vi "handle_websocket_connection.vi"(3 "log queue":refnum<queue>, 4 "remote port":u16, 5 "# conn.":refnum<data-value>, 6 "remote address":string, 7 "quit?":refnum<notifier>, 8 "error in (no error)":errorcluster, 9 "max payload bytes (5012)":i32=5012, 10 "WebSocket Connection Handler":refnum<class "WebSocket Connection Handler.lvclass">, 11 "TCP Network Connection in":refnum<k5>) -> (0 "error out":errorcluster)   [LabVIEW 2019, in "WebSocket Server Toolkit.lvlib"]
uses:
  WebSocket Server Toolkit.lvlib
  types/opcode.ctl
  types/status_code.ctl
  types/frame_data.ctl
  classes/WebSocket Connection Handler/WebSocket Connection Handler.lvclass
  classes/WebSocket Connection/WebSocket Connection.lvclass
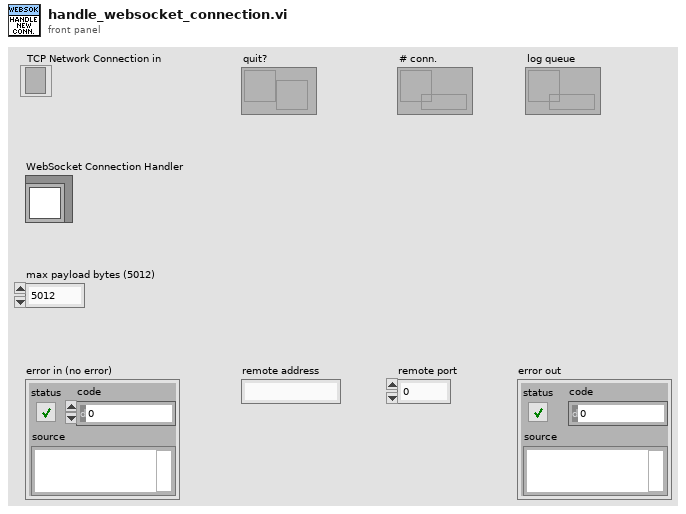
[diagram p1: front panel]
types:
  T1 = typedef "WebSocket Server Toolkit.lvlib/HTTP Request Method.ctl" = enum16{"GET", "HEAD", "POST", "PUT", "DELETE", "CONNECT", "OPTIONS", "TRACE", "PATCH"}
  T2 = typedef "WebSocket Server Toolkit.lvlib/HTTP Protocol Version.ctl" = enum16{"HTTP/0.9", "HTTP/1.0", "HTTP/1.1", "HTTP/2.0", "HTTP/3.0"}
  T3 = typedef "WebSocket Server Toolkit.lvlib/frame_data.ctl" = cluster{"binary?":bool, "frames":string[]}
  T4 = typedef "WebSocket Server Toolkit.lvlib/status_code.ctl" = u16
  T5 = typedef "WebSocket Server Toolkit.lvlib/opcode.ctl" = u8
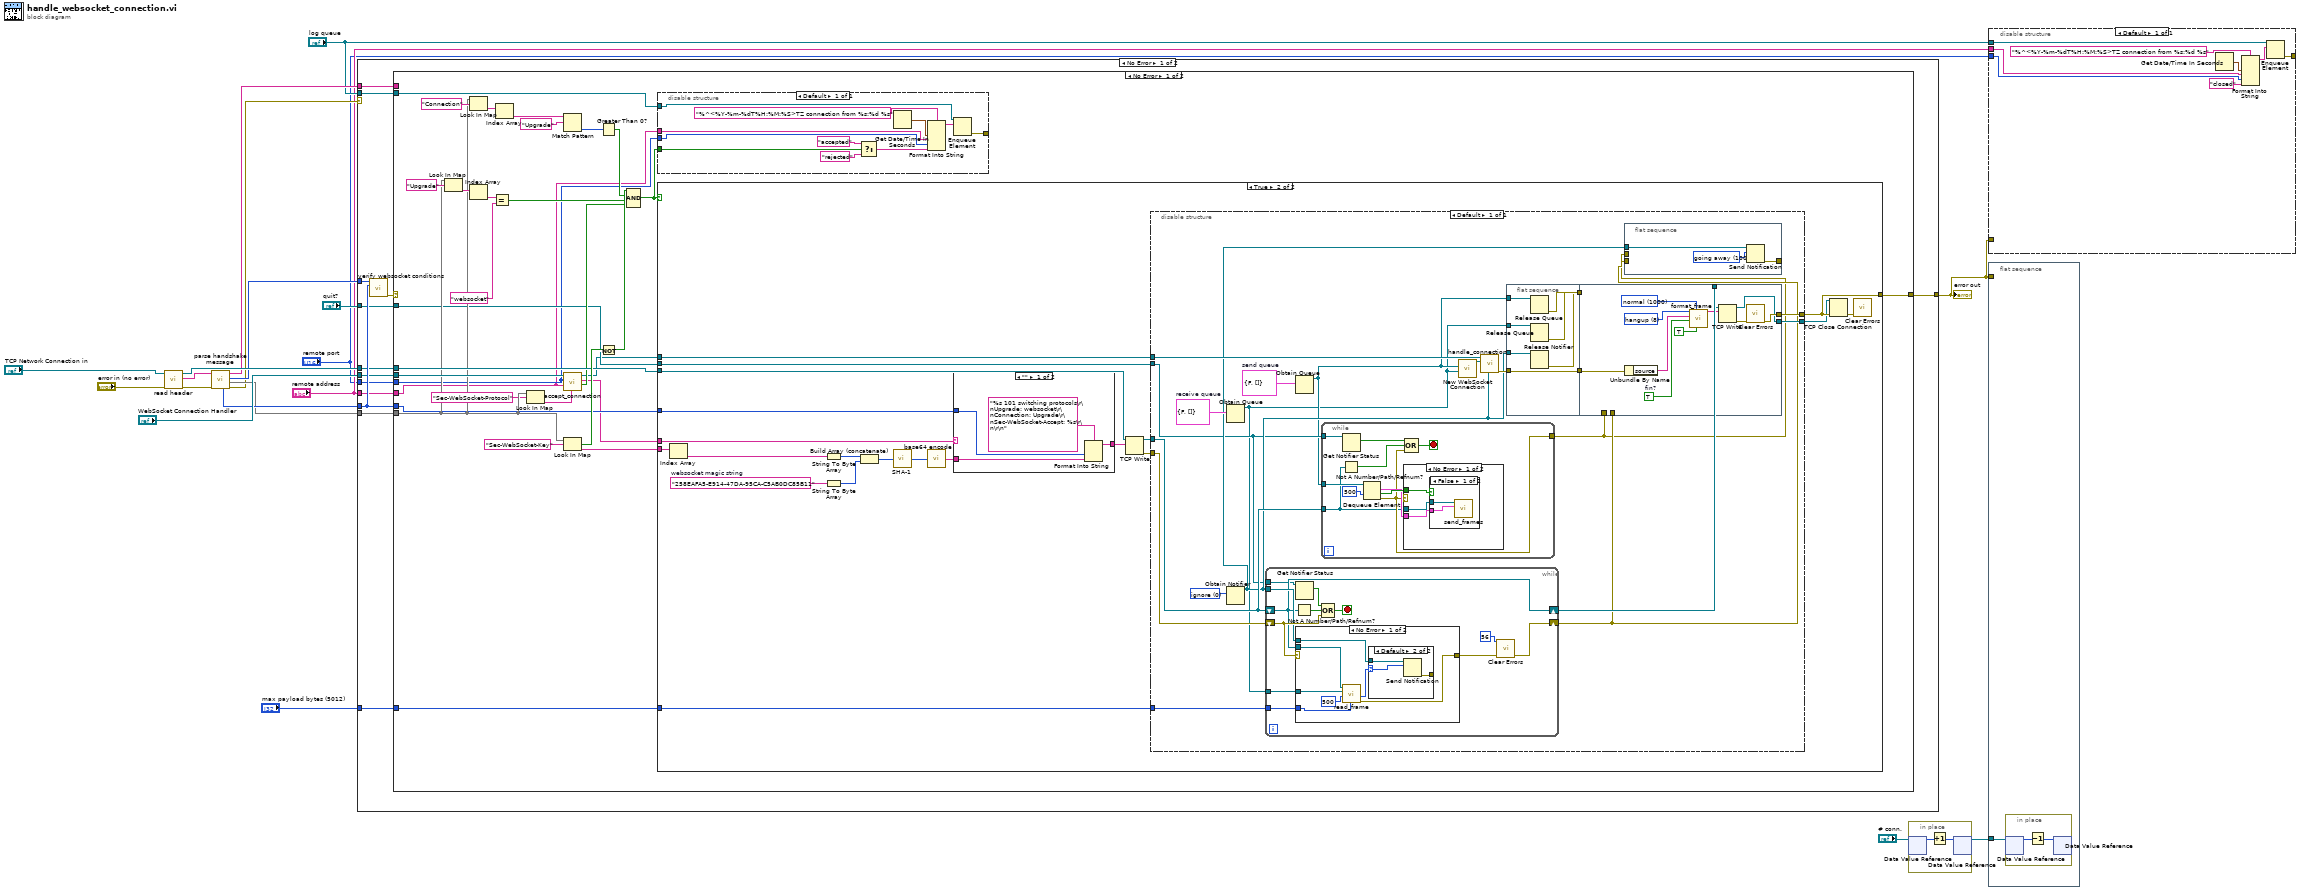
[diagram p0: block diagram]
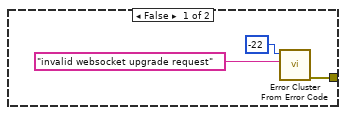
[diagram p2: hidden frame]
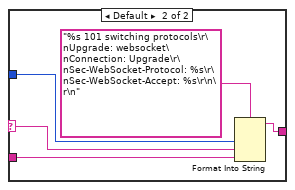
[diagram p7: hidden frame]
diagram:
  n1 = call "read header.vi"("error in (no error)"="error in (no error)", "TCP Network Connection in"="TCP Network Connection in") -> ("error out"=w11:errorcluster, "header content"=w12:string, "TCP Network Connection out"=w18:refnum<k5>)  [unwired: 7 in]
  n2 = call "parse handshake message.vi"("error in"=w11, "String"=w12) -> ("error out"=w13:errorcluster, "headers"=w16:map{string, string[]}, "HTTP method"=w15:T1, "URL"=w14:string, "HTTP protocol version"=w17:T2)  [unwired: 5 in]
  n3 = case shown="No Error" w13 {
    selector: w13 -> [_ w189]
    tunnel: w14 -> [w30 _]
    tunnel: w15 -> [w32 _]
    tunnel: w16 -> [w29 _]
    tunnel: w17 -> [w27 _]
    tunnel: [w28 w189] -> w1
    tunnel: w18 -> [w26 _]
    tunnel: "WebSocket Connection Handler" -> [w25 _]
    tunnel: "remote port" -> [w24 _]
    tunnel: "remote address" -> [w23 _]
    tunnel: "quit?" -> [w22 _]
    tunnel: "max payload bytes (5012)" -> [w21 _]
    tunnel: "log queue" -> [w20 _]
    frame No Error {
      n4 = call "verify websocket conditions.vi"("HTTP protocol version"=w27, "HTTP method"=w32) -> ("error out"=w31:errorcluster)  [unwired: 9 in]
      n5 = case shown="No Error" w31 {
        selector: w31 -> [_ w188]
        tunnel: w30 -> [_ _]
        tunnel: w29 -> [w48 _]
        tunnel: [w53 w188] -> w28
        tunnel: w27 -> [w52 _]
        tunnel: w26 -> [w51 _]
        tunnel: w25 -> [w50 _]
        tunnel: w24 -> [w36 _]
        tunnel: w23 -> [w35 _]
        tunnel: w22 -> [w43 _]
        tunnel: w21 -> [w41 _]
        tunnel: w20 -> [w34 _]
        frame No Error {
          n6 = Look In Map(map=w48, key="Upgrade") -> (value=w59:string[])  [unwired: 1 in, 1 out]
          n7 = Look In Map(map=w48, key="Connection") -> (value=w60:string[])  [unwired: 1 in, 1 out]
          n8 = Index Array(array=w59) -> (element=w49:string)  [unwired: 1 in]
          n9 = Equal?(x=w49, y="websocket") -> (x = y?=w55:bool)
          n10 = Index Array(array=w60) -> (element=w39:string)  [unwired: 1 in]
          n11 = Look In Map(map=w48, key="Sec-WebSocket-Protocol") -> (value=w46:string[])  [unwired: 1 in, 1 out]
          n12 = Match Pattern(string=w39, regular expression="Upgrade" ("y")) -> (offset past match=w38:i32)  [unwired: 1 in, 3 out]
          n13 = call-dynamic "accept_connection.vi"("Sec-WebSocket-Protocol"=w46, "remote address"=w35, "remote port"=w36, "WebSocket Connection Handler in"=w50) -> ("accept connection?"=w45:bool, "Sec-WebSocket-Protocol accepted"=w44:string, "WebSocket Connection Handler out"=w42:refnum<class "WebSocket Connection Handler.lvclass">)  [unwired: 4 in, 1 out]
          n14 = Look In Map(map=w48, key="Sec-WebSocket-Key") -> (key not found?=w57:bool, value=w54:string[])  [unwired: 1 in]
          n15 = Greater Than 0?(x=w38) -> (x > 0?=w37:bool)
          n16 = Not(x=w57) -> (.not. x?=w56:bool)
          n17 = Compound Arithmetic op=AND(w56, w37, w55, w45) -> (w33:bool)
          n18 = disable-structure shown="Default" {
            disable-tunnel: w34 -> [w73]
            disable-tunnel: [w70] -> _
            disable-tunnel: w36 -> [w69]
            disable-tunnel: w35 -> [w68]
            disable-tunnel: w33 -> [w67]
            frame Enabled {
              n19 = Select(t="accepted", s=w67, f="rejected") -> (s? t:f=w64:string)
              n20 = Get Date/Time In Seconds() -> (seconds since 1Jan1904=w71:timestamp)
              n21 = Format Into String(format string="%^<%Y-%m-%dT%H:%M:%S>TZ connection from %s:%d %s", w71, w68, w69, w64) -> (resulting string=w72:string)  [unwired: 2 in, 1 out]
              n22 = Enqueue Element(queue=w73, element=w72) -> (error out=w70:errorcluster)  [unwired: 2 in, 2 out]
            }
          }
          n23 = case shown="True" w33 {
            tunnel: w54 -> [_ w91]
            tunnel: [w75 w85] -> w53
            tunnel: w52 -> [_ w97]
            tunnel: w51 -> [_ w89]
            tunnel: w44 -> [_ w82]
            tunnel: w43 -> [_ w78]
            tunnel: w42 -> [_ w81]
            tunnel: w41 -> [_ w80]
            frame False {
              n24 = call <vilib>:"Error Cluster From Error Code.vi"("error message (\"\")"="invalid websocket upgrade request" ("error message (\"\")"), "error code (0)"=-22) -> ("error out"=w75:errorcluster)  [unwired: 7 in]
            }
            frame True {
              w94 = "258EAFA5-E914-47DA-95CA-C5AB0DC85B11"  # websocket magic string
              n25 = Index Array(array=w91) -> (element=w83:string)  [unwired: 1 in]
              n26 = String To Byte Array(string=w83) -> (unsigned byte array=w92:u8[])
              n27 = String To Byte Array(string=w94) -> (unsigned byte array=w93:u8[])
              n28 = Build Array (concatenate)(w92, w93) -> (w96:u8[])
              n29 = call "SHA-1.vi"("Data"=w96) -> ("message-digest"=w95:u8[])
              n30 = call "base64 encode.vi"("data"=w95) -> ("base64 encoded string"=w90:string)
              n31 = case shown="\"\"" w82 {
                selector: w82 -> [_ w183]
                tunnel: w97 -> [w181 w186]
                tunnel: w90 -> [w180 w184]
                tunnel: [w179 w185] -> w88
                frame "" {
                  n32 = Format Into String(format string="%s 101 switching protocols\r\nUpgrade: websocket\r\nConnection: Upgrade\r\nSec-WebSocket-Accept: %s\r\n\r\n", w181, w180) -> (resulting string=w179:string)  [unwired: 2 in, 1 out]
                }
                frame Default {
                  n33 = Format Into String(format string="%s 101 switching protocols\r\nUpgrade: websocket\nConnection: Upgrade\r\nSec-WebSocket-Protocol: %s\r\nSec-WebSocket-Accept: %s\r\n\r\n", w186, w183, w184) -> (resulting string=w185:string)  [unwired: 2 in, 1 out]
                }
              }
              n34 = TCP Write(connection ID=w89, data in=w88) -> (connection ID out=w87:refnum<k5>, error out=w86:errorcluster)  [unwired: 2 in, 1 out]
              n35 = disable-structure shown="Default" {
                disable-tunnel: w87 -> [w118]
                disable-tunnel: w86 -> [w119]
                disable-tunnel: [w112] -> w85
                disable-tunnel: w81 -> [w117]
                disable-tunnel: w80 -> [w115]
                disable-tunnel: [w111] -> w79
                disable-tunnel: w78 -> [w101]
                frame Enabled {
                  w105 = T3 {"binary?"=FALSE, "frames"=[]}  # receive queue
                  w106 = T3 {"binary?"=FALSE, "frames"=[]}  # send queue
                  w108 = T4 0 items=["ignore"=0, "normal"=1000, "going away"=1001, "protocol error"=1002, "invalid data"=1003] ("status code (ignore)")
                  n36 = Obtain Queue(element data type=w105) -> (queue out=w99:refnum<queue>)  [unwired: 4 in, 2 out]
                  n37 = Obtain Notifier(notification data type=w108) -> (notifier out=w102:refnum<notifier>)  [unwired: 3 in, 2 out]
                  n38 = while {
                    shift-right: [w159] -> w114
                    shift-left: w118 -> [w159]
                    shift-right: [w163] -> w104
                    shift-left: w119 -> [w167]
                    tunnel: w99 -> [w166]
                    tunnel: w115 -> [w164]
                    tunnel: w102 -> [w161]
                    tunnel: w101 -> [w157]
                    stop <- w160 stop-if-true
                    n39 = Not A Number/Path/Refnum?(number/path/refnum=w159) -> (NaN/Path/Refnum?=w158:bool)
                    n40 = Get Notifier Status(notifier=w157) -> (current notification=w156:bool)  [unwired: 1 in, 4 out]
                    n41 = case shown="No Error" w167 {
                      selector: w167 -> [_ w178]
                      tunnel: w159 -> [w174 _]
                      tunnel: w166 -> [w173 _]
                      tunnel: [w171 w178] -> w165
                      tunnel: w164 -> [w170 _]
                      tunnel: w161 -> [w169 _]
                      frame No Error {
                        n42 = call "read_frame.vi"("max payload bytes (5012)"=w170, "timeout ms (500)"=500, "receive queue"=w173, "TCP Network Connection in"=w174) -> ("error out"=w171:errorcluster, "hangup status code (ignore)"=w168:T4)  [unwired: 6 in]
                        n43 = case shown="Default" w168 {
                          selector: w168 -> [_ w175]
                          tunnel: w169 -> [_ w177]
                          tunnel: [_ w176] -> _
                          frame 0 {
                          }
                          frame Default {
                            n44 = Send Notification(notification=w175, notifier=w177) -> (error out=w176:errorcluster)  [unwired: 1 in, 1 out]
                          }
                        }
                      }
                      frame Error {
                      }
                    }
                    n45 = Compound Arithmetic op=OR(w156, w158, w167) -> (w160:bool)
                    n46 = call <vilib>:"Clear Errors.vi"("error in (no error)"=w165, "specific error code to clear (0: all)"=56) -> ("error out"=w163:errorcluster)  [unwired: 4 in, 1 out]
                  }
                  n47 = Obtain Queue(element data type=w106) -> (queue out=w100:refnum<queue>)  [unwired: 4 in, 2 out]
                  n48 = while {
                    tunnel: w100 -> [w150]
                    tunnel: w118 -> [w145]
                    tunnel: [w146] -> w103
                    tunnel: w101 -> [w142]
                    stop <- w144 stop-if-true
                    n49 = Not A Number/Path/Refnum?(number/path/refnum=w145) -> (NaN/Path/Refnum?=w143:bool)
                    n50 = Get Notifier Status(notifier=w142) -> (current notification=w141:bool)  [unwired: 1 in, 4 out]
                    n51 = Dequeue Element(queue=w150, timeout in ms (-1)=500) -> (element=w147:T3, timed out?=w148:bool, error out=w146:errorcluster)  [unwired: 1 in, 1 out]
                    n52 = case shown="No Error" w146 {
                      tunnel: w148 -> [w153 _]
                      tunnel: w147 -> [w152 _]
                      tunnel: w145 -> [w151 _]
                      frame No Error {
                        n53 = case shown="False" w153 {
                          tunnel: w152 -> [w155 _]
                          tunnel: w151 -> [w154 _]
                          frame False {
                            n54 = call "send_frames.vi"("frame data"=w155, "TCP Network Connection in"=w154) -> ()  [unwired: 9 in, 1 out]
                          }
                          frame True {
                          }
                        }
                      }
                      frame Error {
                      }
                    }
                    n55 = Compound Arithmetic op=OR(w141, w143, w146) -> (w144:bool)
                  }
                  n56 = call "New WebSocket Connection.vi"("receive queue"=w99, "send queue"=w100) -> ("WebSocket Connection out"=w98:refnum<class "WebSocket Connection.lvclass">)  [unwired: 8 in, 1 out]
                  n57 = call-dynamic "handle_connection.vi"("hangup?"=w102, "WebSocket Connection"=w98, "WebSocket Connection Handler in"=w117) -> ("error out"=w116:errorcluster)  [unwired: 8 in]
                  n58 = flat-sequence {
                    tunnel: w116 -> [w127]
                    tunnel: w100 -> [w128]
                    tunnel: w99 -> [w129]
                    tunnel: [w127] -> w113
                    tunnel: [w126] -> w110
                    tunnel: [w125] -> w109
                    tunnel: w102 -> [w124]
                    tunnel: [w123] -> w107
                    tunnel: w103 -> [_]
                    tunnel: w104 -> [_]
                    tunnel: w114 -> [w136]
                    tunnel: w113 -> [w133]
                    tunnel: [w131] -> w112
                    tunnel: [w130] -> w111
                    tunnel: w110 -> [_]
                    tunnel: w109 -> [_]
                    tunnel: w107 -> [_]
                    frame #0 {
                      n59 = Release Queue(queue=w128) -> (error out=w125:errorcluster)  [unwired: 2 in, 2 out]
                      n60 = Release Queue(queue=w129) -> (error out=w126:errorcluster)  [unwired: 2 in, 2 out]
                      n61 = Release Notifier(notifier=w124) -> (error out=w123:errorcluster)  [unwired: 2 in, 2 out]
                    }
                    frame #1 {
                      w137 = T4 1000 items=["ignore"=0, "normal"=1000, "going away"=1001, "protocol error"=1002, "invalid data"=1003] ("hangup status code")
                      w140 = TRUE  # fin?
                      w139 = T5 8 items=["continue"=0, "text"=1, "binary"=2, "hangup"=8, "ping"=9, "pong"=10] ("opcode")
                      n62 = Unbundle By Name(w133) -> ("source"=w132:string)
                      n63 = call "format_frame.vi"("mask?"=TRUE, "hangup status code"=w137, "fin?"=w140, "data in"=w132, "opcode"=w139) -> ("frame data out"=w135:string)  [unwired: 6 in]
                      n64 = TCP Write(connection ID=w136, data in=w135) -> (connection ID out=w130:refnum<k5>, error out=w134:errorcluster)  [unwired: 2 in, 1 out]
                      n65 = call <vilib>:"Clear Errors.vi"("error in (no error)"=w134) -> ("error out"=w131:errorcluster)  [unwired: 5 in, 1 out]
                    }
                  }
                  n66 = flat-sequence {
                    tunnel: w104 -> [_]
                    tunnel: w103 -> [_]
                    tunnel: w102 -> [w122]
                    tunnel: [w120] -> _
                    frame #0 {
                      w121 = T4 1001 items=["ignore"=0, "normal"=1000, "going away"=1001, "protocol error"=1002, "invalid data"=1003] ("notification")
                      n67 = Send Notification(notification=w121, notifier=w122) -> (error out=w120:errorcluster)  [unwired: 1 in, 1 out]
                    }
                  }
                }
              }
              n68 = TCP Close Connection(connection ID=w79, error in (no error)=w85) -> (error out=w84:errorcluster)  [unwired: 1 in, 1 out]
              n69 = call <vilib>:"Clear Errors.vi"("error in (no error)"=w84) -> ()  [unwired: 5 in, 2 out]
            }
          }
        }
        frame Error {
        }
      }
    }
    frame Error {
    }
  }
  "error out" <- w1
  n70 = in-place {
    n71 = in-place-dvr #1("# conn.") -> (w191:u32)  [unwired: 1 out]
    n72 = Increment(x=w191) -> (x+1=w190:u32)
    n73 = in-place-dvr #1(w190) -> (w5:refnum<data-value>)  [unwired: 1 out]
  }
  n74 = disable-structure shown="Default" {
    disable-tunnel: "log queue" -> [w198]
    disable-tunnel: [w195] -> _
    disable-tunnel: "remote port" -> [w194]
    disable-tunnel: "remote address" -> [w193]
    disable-tunnel: w1 -> [_]
    frame Enabled {
      n75 = Get Date/Time In Seconds() -> (seconds since 1Jan1904=w196:timestamp)
      n76 = Format Into String(format string="%^<%Y-%m-%dT%H:%M:%S>TZ connection from %s:%d %s", w196, w193, w194, "closed") -> (resulting string=w197:string)  [unwired: 2 in, 1 out]
      n77 = Enqueue Element(queue=w198, element=w197) -> (error out=w195:errorcluster)  [unwired: 2 in, 2 out]
    }
  }
  n78 = flat-sequence {
    tunnel: w5 -> [w200]
    tunnel: w1 -> [_]
    frame #0 {
      n79 = in-place {
        n80 = in-place-dvr #2(w200) -> (w202:u32)  [unwired: 1 out]
        n81 = Decrement(x=w202) -> (x-1=w201:u32)
        n82 = in-place-dvr #2(w201) -> ()  [unwired: 2 out]
      }
    }
  }
